vi "LV to ITX Retrieve.vi"(0 "File or Folder Path":path=path "C:/", 5 "offset":i32, 7 "length":i32=1, 9 "index":T2={"A"=1, "B"=0, "C"=2, "D"=0, "E"=3, "N1"=0, "N2"=0, "N3"=0, "N4"=0}) -> (4 "A vs B":cluster{dbl[], dbl[]}[](graph), 6 "C vs D":cluster{dbl[], dbl[]}[](graph), 8 "E":dbl[][](graph), 10 "N":cluster{"N1":dbl, "N2":dbl, "N3":dbl, "N4":dbl}={"N1"=0.0624995231628418, "N2"=0.0624995231628418, "N3"=0.0624995231628418, "N4"=0.0624995231628418} {"N4" format="%#_6p"; "N3" format="%#_6p"; "N2" format="%#_6p"; "N1" format="%#_6p"}, 14 "Comments":string)   [LabVIEW 2016, in "LVtoITX.lvclass"]
uses:
  LVtoITX.lvclass
  <vilib>/Utility/miscctls.llb/LVOffsetAndMultiplierTypeDef.ctl
  Typedefs/Retrieve Data Type.ctl
panel:
  in  "DAT header length":i32=11
  in  "Data Type":T1=enum."DAT"
  in  "D  is time?":bool
  in  "B is time?":bool
  out "time":string[][](table)
  in  "Use Folder Index File?":bool
  in  "Generate Folder Index File?":bool
  in  "Ez name":string="Ez name"
  in  "Ey name":string="Ey name"
  in  "Ex name":string="Ex name"
  in  "C y name":string="C y name"
  in  "D x name":string="D x name"
  in  "A y name":string="A y name"
  in  "B x name":string="B x name"
  out "Index, Wavenames":string[][](table)
  in  "recolor traces?":bool
  in  "Ex":T3={"Offset"=0.0, "Multiplier"=1.0}
  in  "Ey":T3={"Offset"=0.0, "Multiplier"=1.0}
  out "Path":path
  out "counter":i32
  out "pattern":string="*.dat"
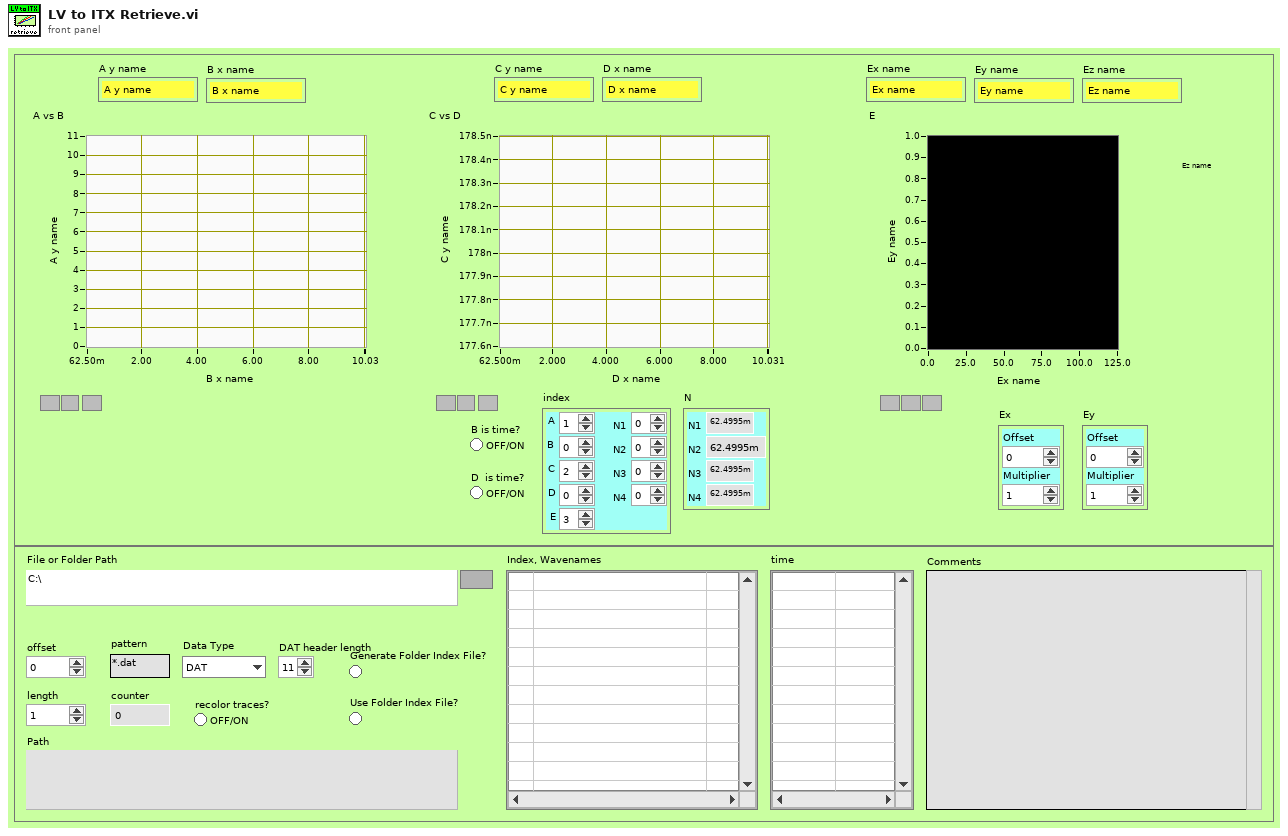
[diagram p1: front panel]
types:
  T1 = typedef "LVtoITX.lvclass/Retrieve Data Type.ctl" = enum16{"ITX", "ITX w/ 2D", "DAT"}
  T2 = cluster{"A":i32, "B":i32, "C":i32, "D":i32, "E":i32, "N1":i32, "N2":i32, "N3":i32, "N4":i32}
  T3 = typedef "LVOffsetAndMultiplierTypeDef.ctl" = cluster{"Offset":dbl, "Multiplier":dbl}
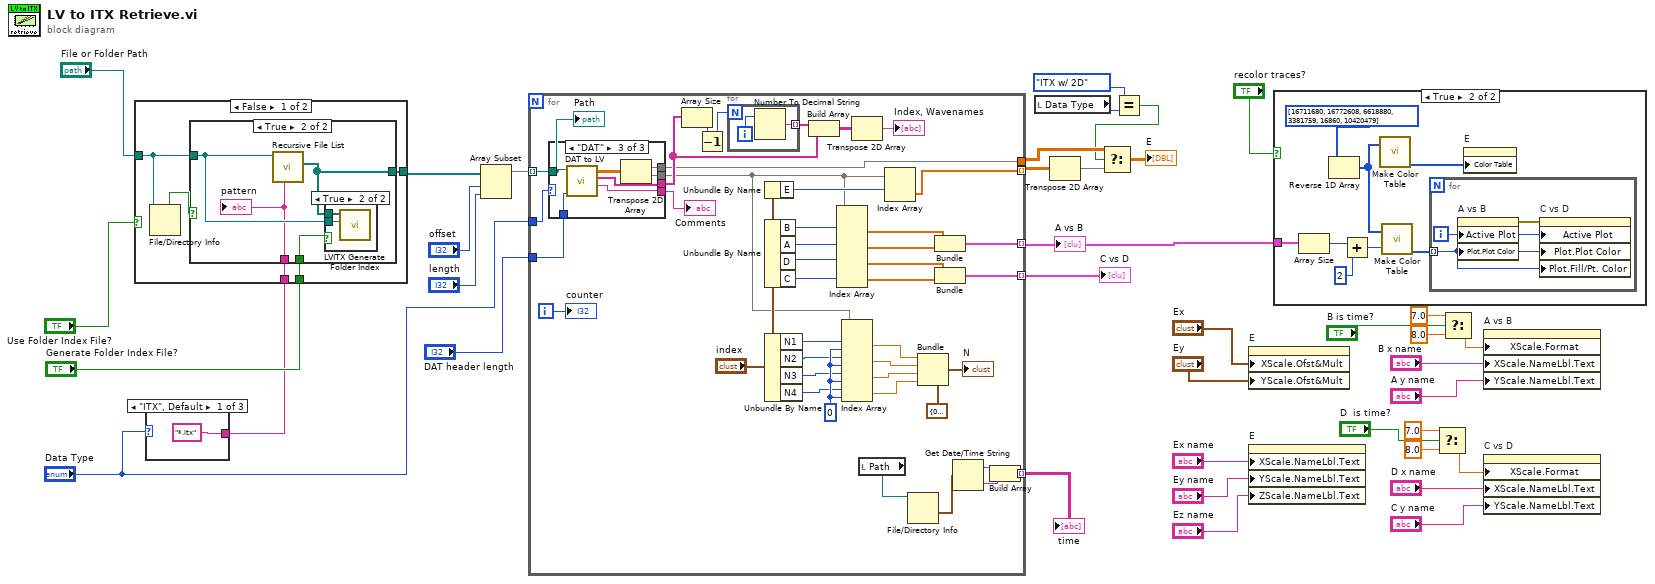
[diagram p0: block diagram]
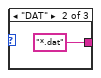
[diagram p2: hidden frame]
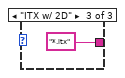
[diagram p3: hidden frame]
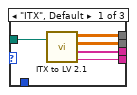
[diagram p5: hidden frame]
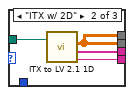
[diagram p6: hidden frame]
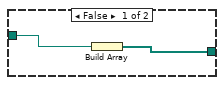
[diagram p7: hidden frame]
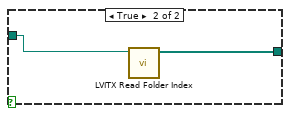
[diagram p9: hidden frame]
diagram:
  n1 = case shown="\"ITX\", Default" "Data Type" {
    tunnel: ["*.itx" ("pattern") "*.dat" ("pattern") "*.itx" ("pattern")] -> w1
    frame "ITX", Default {
    }
    frame "DAT" {
    }
    frame "ITX w/ 2D" {
    }
  }
  n2 = case shown="False" "Use Folder Index File?" {
    tunnel: [w44 w55] -> w36
    tunnel: "File or Folder Path" -> [w46 w56]
    tunnel: "Generate Folder Index File?" -> [w43 _]
    tunnel: w1 -> [w42 _]
    frame False {
      n3 = File/Directory Info(path=w46) -> (directory=w45:bool)  [unwired: 1 in, 6 out]
      n4 = case shown="True" w45 {
        tunnel: [w48 w50] -> w44
        tunnel: w46 -> [w47 w52]
        tunnel: w43 -> [_ w51]
        tunnel: w42 -> [_ w49]
        frame False {
          n5 = Build Array(w47) -> (w48:path[])
        }
        frame True {
          n6 = call <vilib>:"Recursive File List.vi"("pattern"=w49, "Folder Path"=w52) -> ("All Files in Dir"=w50:path[])  [unwired: 5 in, 4 out]
          n7 = case shown="True" w51 {
            tunnel: w50 -> [_ w54]
            tunnel: w52 -> [_ w53]
            frame False {
            }
            frame True {
              n8 = call "LVITX Generate Folder Index.vi"("File or Folder Path"=w53, "All Files in Dir"=w54) -> ()  [unwired: 10 in]
            }
          }
          "pattern" <- w49
        }
      }
    }
    frame True {
      n9 = call "LVITX Read Folder Index.vi"("File or Folder Path"=w56) -> ("Array"=w55:path[])  [unwired: 10 in]
    }
  }
  n10 = Array Subset(array=w36, index="offset", length="length") -> (w15:path[])
  n11 = for {
    tunnel: w15 -> [w96] mode=indexing
    tunnel: [w96] -> _ mode=indexing
    tunnel: [w95] -> w27 mode=indexing
    tunnel: [w94] -> w26 mode=indexing
    tunnel: [w71] -> w31 mode=indexing
    tunnel: [w85] -> w29
    tunnel: [w60] -> w18 mode=indexing
    tunnel: "Data Type" -> [w58]
    tunnel: "DAT header length" -> [w57]
    i -> [w98]
    w84 = 0 ("disabled index (col)")
    n12 = case shown="\"DAT\"" w58 {
      tunnel: [w103 w109 w113] -> w97
      tunnel: [w104 w107 w110] -> w63
      tunnel: w96 -> [w105 w108 w115]
      tunnel: [w102 w106 w112] -> w86
      tunnel: [w101 w107 w110] -> w85
      tunnel: w57 -> [_ _ w114]
      frame "ITX", Default {
        n13 = call "ITX to LV 2.1.vi"("file (use dialog)"=w105) -> ("2D array"=w101:dbl[][], "1D arrays"=w104:dbl[][], "wave names"=w102:string[], "Notes"=w103:string)  [unwired: 1 in]
      }
      frame "ITX w/ 2D" {
        n14 = call "ITX to LV 2.1 1D.vi"("file (use dialog)"=w108) -> ("1D arrays"=w107:dbl[][], "wave names"=w106:string[], "Notes"=w109:string)  [unwired: 2 in]
      }
      frame "DAT" {
        n15 = call "DAT to LV.vi"("header length"=w114, "File Path"=w115) -> ("Comments"=w113:string, "Wavenames"=w112:string[], "Data"=w111:dbl[][])  [unwired: 7 in]
        n16 = Transpose 2D Array(2D array=w111) -> (transposed array=w110:dbl[][])
      }
    }
    "Comments" <- w97
    n17 = Array Size(array=w86) -> (size(s)=w89:i32)
    n18 = Decrement(x=w89) -> (x-1=w88:i32)
    n19 = for {
      N: w88 -> [_]
      tunnel: [w99] -> w92 mode=indexing
      i -> [w100]
      n20 = Number To Decimal String(number=w100) -> (decimal integer string=w99:string)  [unwired: 1 in]
    }
    n21 = Unbundle By Name("index") -> ("E"=w76:i32)
    n22 = Unbundle By Name("index") -> ("B"=w75:i32, "A"=w74:i32, "D"=w73:i32, "C"=w72:i32)
    n23 = Unbundle By Name("index") -> ("N1"=w77:i32, "N2"=w78:i32, "N3"=w79:i32, "N4"=w80:i32)
    n24 = Build Array(w92, w86) -> (w87:string[][])
    n25 = Index Array(array=w63, index (row) #1=w75, index (row) #2=w74, index (row) #3=w73, index (row) #4=w72) -> (element #1=w68:dbl[], element #2=w67:dbl[], element #3=w90:dbl[], element #4=w93:dbl[])  [unwired: 4 in]
    n26 = Index Array(array=w63, index (row) #1=w77, index (col) #1=w84, index (row) #2=w78, index (col) #2=w84, index (row) #3=w79, index (col) #3=w84, index (row) #4=w80, index (col) #4=w84) -> (element #1=w64:dbl, element #2=w65:dbl, element #3=w66:dbl, element #4=w83:dbl)
    n27 = Transpose 2D Array(2D array=w87) -> (transposed array=→"Index, Wavenames":string[][])
    n28 = local read "Path"() -> (w69:path)
    n29 = Index Array(array=w63, index (row)=w76) -> (element=w71:dbl[])  [unwired: 1 in]
    n30 = File/Directory Info(path=w69) -> (last mod=w59:timestamp)  [unwired: 1 in, 6 out]
    n31 = Bundle(cluster=cluster{"N1":dbl, "N2":dbl, "N3":dbl, "N4":dbl} {"N1"=0.0, "N2"=0.0, "N3"=0.0, "N4"=0.0}, "N1"=w64, "N2"=w65, "N3"=w66, "N4"=w83) -> (→"N":cluster{"N1":dbl, "N2":dbl, "N3":dbl, "N4":dbl})
    n32 = Bundle("1D arrays"=w68, "1D arrays"=w67) -> (w95:cluster{"1D arrays":dbl[], "1D arrays":dbl[]})  [unwired: 1 in]
    n33 = Bundle("1D arrays"=w90, "1D arrays"=w93) -> (w94:cluster{"1D arrays":dbl[], "1D arrays":dbl[]})  [unwired: 1 in]
    n34 = Get Date/Time String(seconds (now)=w59) -> (date string=w62:string, time string=w61:string)  [unwired: 2 in]
    n35 = Build Array(w62, w61) -> (w60:string[])
    "counter" <- w98
    "Path" <- w96
  }
  "A vs B" <- w27
  "C vs D" <- w26
  "time" <- w18
  n36 = local read "Data Type"() -> (w5:T1)
  n37 = Transpose 2D Array(2D array=w31) -> (transposed array=w32:dbl[][])
  n38 = Equal?(x=enum16{"ITX", "ITX w/ 2D", "DAT"}."ITX w/ 2D" ("Enum"), y=w5) -> (x = y?=w3:bool)
  n39 = Select(t=w29, s=w3, f=w32) -> (s? t:f=→"E":dbl[][])
  n40 = property on="E" class="IntGraph (strict)"("XScale.Ofst&Mult"="Ex", "YScale.Ofst&Mult"="Ey") -> ()  [unwired: 2 in, 2 out]
  n41 = property on="E" class="IntGraph (strict)"("XScale.NameLbl.Text"="Ex name", "YScale.NameLbl.Text"="Ey name", "ZScale.NameLbl.Text"="Ez name") -> ()  [unwired: 2 in, 2 out]
  n42 = case shown="True" "recolor traces?" {
    tunnel: w27 -> [_ w118]
    frame False {
    }
    frame True {
      n43 = Array Size(array=w118) -> (size(s)=w119:i32)
      n44 = Reverse 1D Array(array=u32[] [16711680, 16772608, 6618880, 3381759, 16860, 10420479] ("color scale")) -> (reversed array=w117:u32[])
      n45 = Add(x=w119, y=2 ("x")) -> (x+y=w123:i32)
      n46 = call <userlib>:"Make Color Table.vi"("Array"=w117) -> ("Color Tbl"=w121:u32[])  [unwired: 1 in, 3 out]
      n47 = call <userlib>:"Make Color Table.vi"("Array"=w117, "Size/3"=w123) -> ("Color Tbl"=w120:u32[])  [unwired: 3 out]
      n48 = for {
        tunnel: w120 -> [w124] mode=indexing
        i -> [w125]
        n49 = property on="A vs B" class="XYGraph (strict)"("Active Plot"=w125, "Plot.Plot Color"=w124) -> (error out=w126:errorcluster)  [unwired: 2 in, 1 out]
        n50 = property on="C vs D" class="XYGraph (strict)"(error in=w126, "Active Plot"=w125, "Plot.Plot Color"=w124, "Plot.Fill/Pt. Color"=w124) -> ()  [unwired: 1 in, 2 out]
      }
      n51 = property on="E" class="IntGraph (strict)"("Color Table"=w121) -> ()  [unwired: 2 in, 2 out]
    }
  }
  n52 = Select(t=7.0, s="D  is time?", f=8.0) -> (s? t:f=w11:dbl)
  n53 = Select(t=7.0, s="B is time?", f=8.0) -> (s? t:f=w12:dbl)
  n54 = property on="A vs B" class="XYGraph (strict)"("XScale.Format"=w12, "XScale.NameLbl.Text"="B x name", "YScale.NameLbl.Text"="A y name") -> ()  [unwired: 2 in, 2 out]
  n55 = property on="C vs D" class="XYGraph (strict)"("XScale.Format"=w11, "XScale.NameLbl.Text"="D x name", "YScale.NameLbl.Text"="C y name") -> ()  [unwired: 2 in, 2 out]
